vi "IVI DC Power Supply Initialization VI.vi"(8 "error in (no error)":errorcluster, 10 "Custom XML":string, 11 "Device Item Ref in":T3 format="%.0x") -> (0 "error out":errorcluster, 3 "Device Item Ref out":T3 format="%.0x")   [LabVIEW 2011, in "IVI DC Power Supply Custom Device.lvlib"]
uses:
  IVI DC Power Supply Custom Device.lvlib
  <vilib>/NI Veristand/Custom Device API/Custom Device Item Ref.ctl
  <vilib>/NI Veristand/Custom Device API/Custom Device Channel.ctl
  <vilib>/NI Veristand/Custom Device API/Custom Device Channel Type.ctl
  Global.vi
  <vilib>/NI Veristand/Custom Device API/Custom Device API.lvlib
panel:
  in  "Output Channels":T1={"Type"=enum."Output", "Units"="", "Default Value"=0.0, "Faultable"=FALSE, "Scalable"=FALSE}
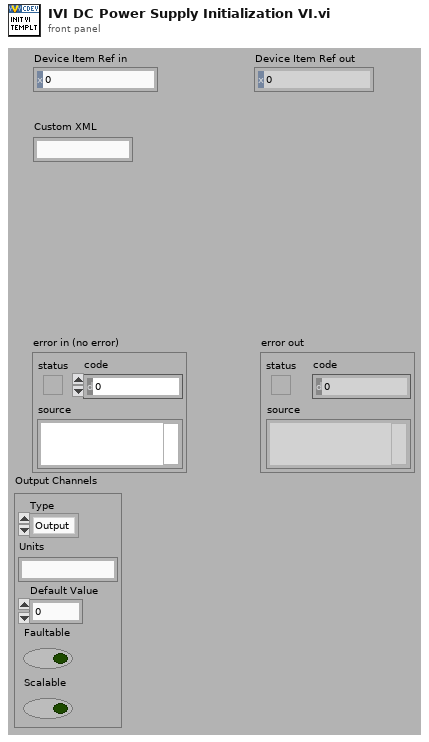
[diagram p1: front panel]
types:
  T1 = typedef "Custom Device API.lvlib/Custom Device Channel.ctl" = cluster{"Type":T2, "Units":string, "Default Value":dbl, "Faultable":bool, "Scalable":bool}
  T2 = typedef "Custom Device API.lvlib/Custom Device Channel Type.ctl" = enum16{"Input", "Output"}
  T3 = typedef "Custom Device API.lvlib/Custom Device Item Ref.ctl" = u64
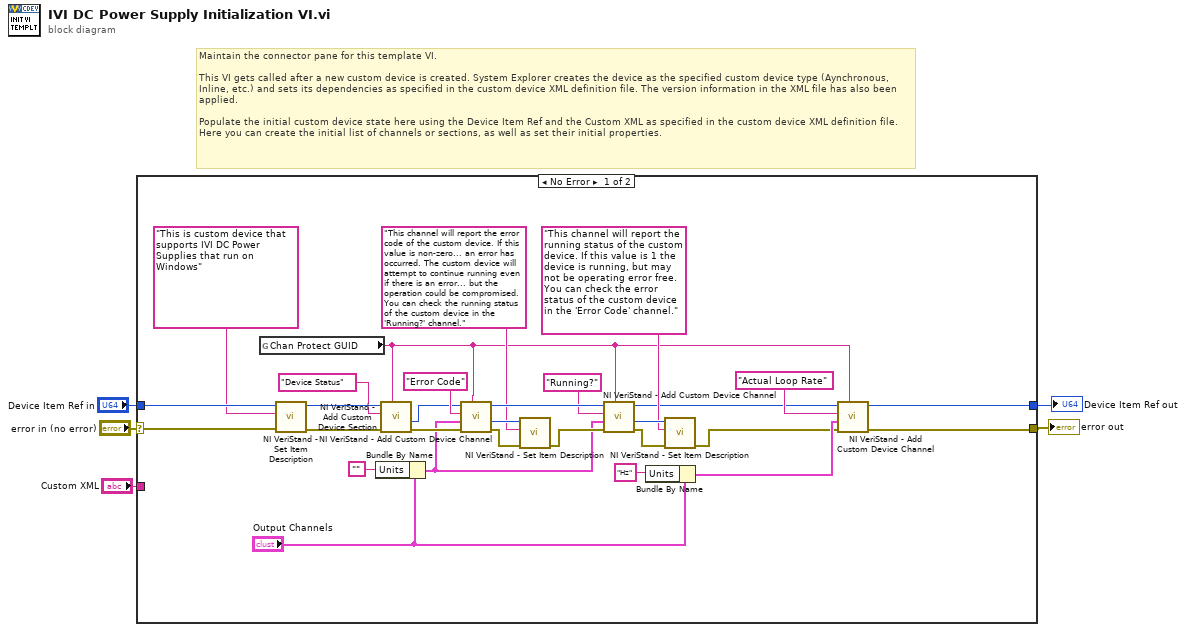
[diagram p0: block diagram]
diagram:
  # "Maintain the connector pane for this template VI.\n\nThis VI gets called after a new custom device is created. System Explorer creates the device as the specified custom device type (Aynchronous, Inline, etc.) and sets its dependencies as specified in the custom device XML definition file. The version information in the XML file has also been applied.\n\nPopulate the initial custom device state here using the Device Item Ref and the Custom XML as specified in the custom device XML definition file. Here you can create the initial list of channels or sections, as well as set their initial properties."
  n1 = case shown="No Error" "error in (no error)" {
    selector: "error in (no error)" -> [w34 w35]
    tunnel: "Device Item Ref in" -> [w33 w36]
    tunnel: "Custom XML" -> [_ _]
    tunnel: [w11 w36] -> w1
    tunnel: [w12 w35] -> w2
    frame No Error {
      n2 = global read "Global.vi" "Chan Protect GUID"() -> (w6:string)
      n3 = call <vilib>:"NI VeriStand - Set Item Description.vi"("error in (no error)"=w34, "Description"="This is custom device that supports IVI DC Power Supplies that run on Windows", "Item Ref in"=w33) -> ("error out"=w32:errorcluster, "Item Ref out"=w31:T3)  [unwired: 6 in, 1 out]
      n4 = Bundle By Name(cluster="Output Channels", "Units"="") -> (w18:T1)
      n5 = call <vilib>:"NI VeriStand - Add Custom Device Section.vi"("GUID (Default Section)"=w6, "error in (no error)"=w32, "Section Name"="Device Status", "Parent Ref in"=w31) -> ("error out"=w29:errorcluster, "Section Ptr"=w15:T3)  [unwired: 4 in, 2 out]
      n6 = call <vilib>:"NI VeriStand - Add Custom Device Channel.vi"("GUID (Default Channel)"=w6, "error in (no error)"=w29, "Channel"=w18, "Channel Name"="Error Code", "Parent Ref in"=w15) -> ("error out"=w26:errorcluster, "Channel Ref"=w27:T3, "Parent Ref out"=w25:T3)  [unwired: 3 in, 1 out]
      n7 = call <vilib>:"NI VeriStand - Set Item Description.vi"("error in (no error)"=w26, "Description"="This channel will report the error code of the custom device. If this value is non-zero... an error has occurred. The custom device will attempt to continue running even if there is an error... but the operation could be compromised. You can check the running status of the custom device in the 'Running?' channel.", "Item Ref in"=w27) -> ("error out"=w24:errorcluster)  [unwired: 6 in, 2 out]
      n8 = call <vilib>:"NI VeriStand - Add Custom Device Channel.vi"("GUID (Default Channel)"=w6, "error in (no error)"=w24, "Channel"=w18, "Channel Name"="Running?", "Parent Ref in"=w25) -> ("error out"=w22:errorcluster, "Channel Ref"=w21:T3, "Parent Ref out"=w8:T3)  [unwired: 3 in, 1 out]
      n9 = Bundle By Name(cluster="Output Channels", "Units"="Hz") -> (w9:T1)
      n10 = call <vilib>:"NI VeriStand - Set Item Description.vi"("error in (no error)"=w22, "Description"="This channel will report the running status of the custom device. If this value is 1 the device is running, but may not be operating error free.  You can check the error status of the custom device in the 'Error Code' channel.", "Item Ref in"=w21) -> ("error out"=w7:errorcluster)  [unwired: 6 in, 2 out]
      n11 = call <vilib>:"NI VeriStand - Add Custom Device Channel.vi"("GUID (Default Channel)"=w6, "error in (no error)"=w7, "Channel"=w9, "Channel Name"="Actual Loop Rate", "Parent Ref in"=w8) -> ("error out"=w12:errorcluster, "Parent Ref out"=w11:T3)  [unwired: 3 in, 2 out]
    }
    frame Error {
    }
  }
  "error out" <- w2
  "Device Item Ref out" <- w1
